vi "Autonomous Independent.vi"   [LabVIEW 2019]
doc: "This VI is called when autonomous begins, and will automatically be terminated when autonomous ends. You can carry out timed or sensor driven robot movement independently without needing to return to the caller."
uses:
  Robot Global Data.vi
  <vilib>/Rock Robotics/Network Tables/NT Read String.vi
panel:
  # "Be sure to right-click and choose Data Operations>>Make Current Value default if you want to save the array values with the VI"
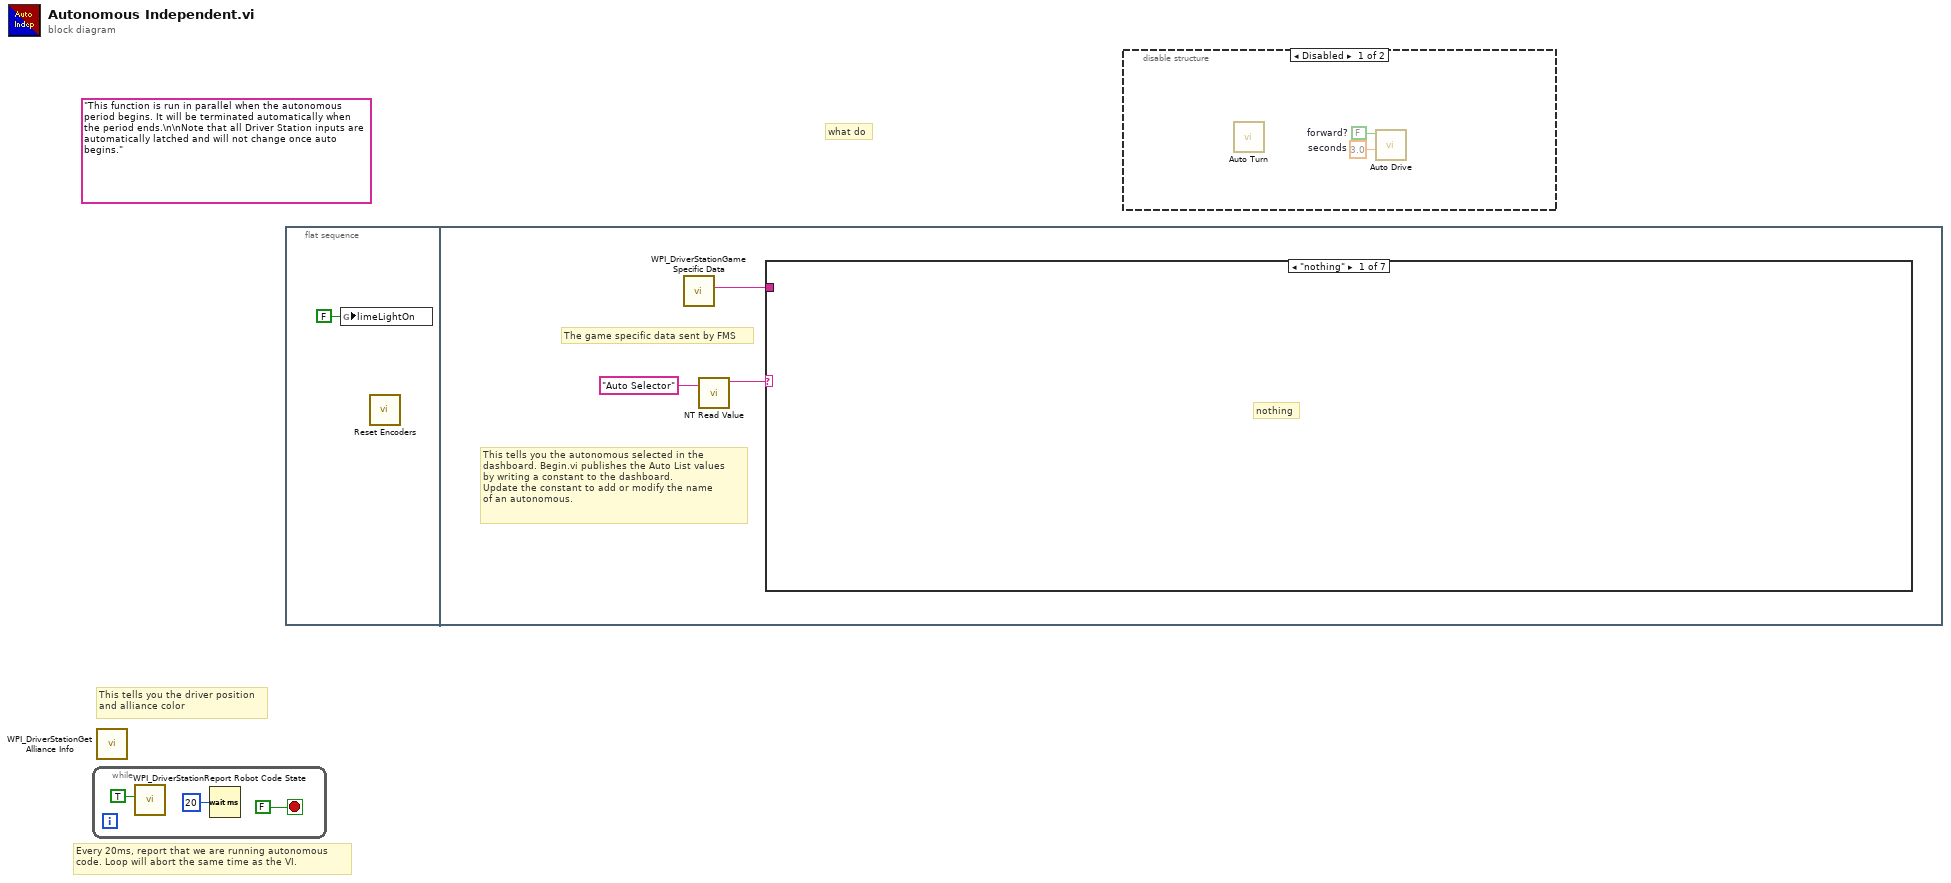
[diagram p0: block diagram]
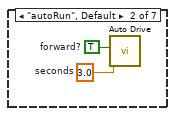
[diagram p3: hidden frame]
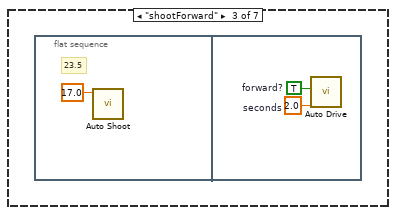
[diagram p4: hidden frame]
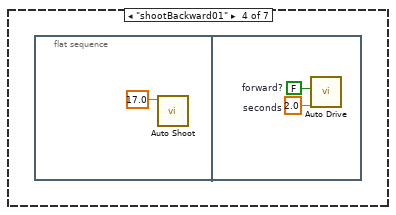
[diagram p5: hidden frame]
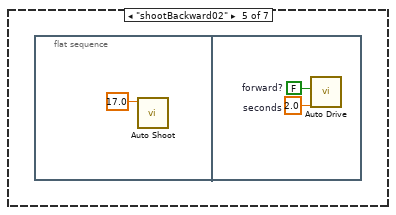
[diagram p6: hidden frame]
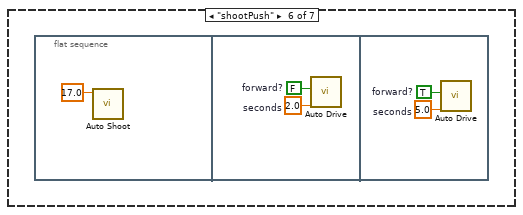
[diagram p7: hidden frame]
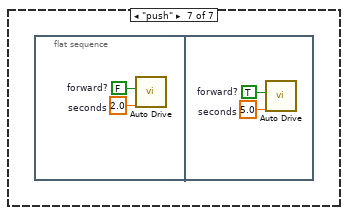
[diagram p8: hidden frame]
diagram:
  (unwired) "This function is run in parallel when the autonomous period begins. It will be terminated automatically when the period ends.\n\nNote that all Driver Station inputs are automatically latched and will not change once auto begins."
  # "what do"
  # "Every 20ms, report that we are running autonomous\ncode. Loop will abort the same time as the VI."
  # "This tells you the driver position\nand alliance color"
  n1 = while {
    stop <- FALSE stop-if-true
    n2 = call <vilib>:"WPI_DriverStationReport Robot Code State.vi"("Autonomous"=TRUE) -> ()  [unwired: 10 in, 1 out]
    n3 = Wait (ms)(milliseconds to wait=u32 20) -> ()  [unwired: 1 out]
  }
  n4 = call <vilib>:"WPI_DriverStationGet Alliance Info.vi"() -> ()  [unwired: 12 out]
  n5 = flat-sequence {
    frame #0 {
      n6 = global write "Robot Global Data.vi" "limeLightOn"(FALSE ("limeLightOn")) -> ()
      n7 = call "Reset Encoders.vi"() -> ()  [unwired: 12 in]
    }
    frame #1 {
      # "The game specific data sent by FMS"
      # "This tells you the autonomous selected in the \ndashboard. Begin.vi publishes the Auto List values\nby writing a constant to the dashboard.\nUpdate the constant to add or modify the name\nof an autonomous."
      n8 = call <vilib>:"WPI_DriverStationGame Specific Data.vi"() -> ("Game Specific Data"=w5:string)  [unwired: 11 in]
      n9 = call-poly <vilib>:"NT Read Value.vi"("Name"="Auto Selector") -> ("String"=w6:string)  [unwired: 9 in, 1 out]
      n10 = case shown="\"nothing\"" w6 {
        tunnel: w5 -> [_ _ _ _ _ _ _]
        frame "nothing" {
          # "nothing"
        }
        frame "autoRun", Default {
          w8 = 3.0  # seconds
          w9 = TRUE  # forward?
          n11 = call "Auto Drive.vi"("seconds"=w8, "forward?"=w9) -> ()  [unwired: 10 in]
        }
        frame "shootForward" {
          n12 = flat-sequence {
            frame #0 {
              # "23.5"
              n13 = call "Auto Shoot.vi"("angle"=17.0) -> ()  [unwired: 11 in]
            }
            frame #1 {
              w11 = 2.0  # seconds
              w12 = TRUE  # forward?
              n14 = call "Auto Drive.vi"("seconds"=w11, "forward?"=w12) -> ()  [unwired: 10 in]
            }
          }
        }
        frame "shootBackward01" {
          n15 = flat-sequence {
            frame #0 {
              n16 = call "Auto Shoot.vi"("angle"=17.0) -> ()  [unwired: 11 in]
            }
            frame #1 {
              w14 = 2.0  # seconds
              w15 = FALSE  # forward?
              n17 = call "Auto Drive.vi"("seconds"=w14, "forward?"=w15) -> ()  [unwired: 10 in]
            }
          }
        }
        frame "shootBackward02" {
          n18 = flat-sequence {
            frame #0 {
              n19 = call "Auto Shoot.vi"("angle"=17.0) -> ()  [unwired: 11 in]
            }
            frame #1 {
              w17 = 2.0  # seconds
              w18 = FALSE  # forward?
              n20 = call "Auto Drive.vi"("seconds"=w17, "forward?"=w18) -> ()  [unwired: 10 in]
            }
          }
        }
        frame "shootPush" {
          n21 = flat-sequence {
            frame #0 {
              n22 = call "Auto Shoot.vi"("angle"=17.0) -> ()  [unwired: 11 in]
            }
            frame #1 {
              w20 = 2.0  # seconds
              w21 = FALSE  # forward?
              n23 = call "Auto Drive.vi"("seconds"=w20, "forward?"=w21) -> ()  [unwired: 10 in]
            }
            frame #2 {
              w23 = 5.0  # seconds
              w22 = TRUE  # forward?
              n24 = call "Auto Drive.vi"("seconds"=w23, "forward?"=w22) -> ()  [unwired: 10 in]
            }
          }
        }
        frame "push" {
          n25 = flat-sequence {
            frame #0 {
              w24 = 2.0  # seconds
              w25 = FALSE  # forward?
              n26 = call "Auto Drive.vi"("seconds"=w24, "forward?"=w25) -> ()  [unwired: 10 in]
            }
            frame #1 {
              w27 = 5.0  # seconds
              w26 = TRUE  # forward?
              n27 = call "Auto Drive.vi"("seconds"=w27, "forward?"=w26) -> ()  [unwired: 10 in]
            }
          }
        }
      }
    }
  }
  n28 = disable-structure shown="Disabled" {
    frame Disabled {
      w28 = FALSE  # forward?
      w29 = 3.0  # seconds
      n29 = call "Auto Turn.vi"() -> ()  [unwired: 12 in]
      n30 = call "Auto Drive.vi"("seconds"=w29, "forward?"=w28) -> ()  [unwired: 10 in]
    }
    frame Enabled {
    }
  }
